vi "BackupPeriodicTasks.vi"() -> ()   [LabVIEW 2014]
uses:
  <vilib>/Rock Robotics/WPI/Joystick/WPI_JoystickGetSetRefNum.vi
  SwerveCode/SteerGlobals.vi
  <vilib>/addons/control/pid/pid.llb/PID (DBL).vi
  <vilib>/addons/control/pid/NI_PID_pid.lvlib
panel:
  in  "PID gains":T1={"proportional gain (Kc)"=0.0017, "integral time (Ti, min)"=0.01, "derivative time (Td, min)"=0.00173} {"derivative time (Td, min)" format="%.5f"; "integral time (Ti, min)" format="%.3f"; "proportional gain (Kc)" format="%.5f"}
  in  "error in":errorcluster
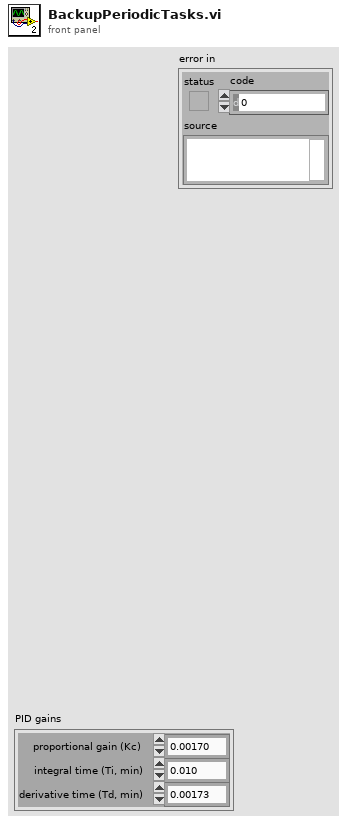
[diagram p1: front panel]
types:
  T1 = cluster{"proportional gain (Kc)":dbl, "integral time (Ti, min)":dbl, "derivative time (Td, min)":dbl}
  T2 = typedef "WPI_MotorControlDeviceRef.ctl" = cluster{"DeviceStatus":errorcluster, "Type":T3, "PWM":cluster{"Controller":T4, "PWM Channel":T5, "DeadBand":T6}, "CAN":cluster{"Device Number":u8, "Control Mode":T7, "Semaphore":T8, "Max Vout":dbl, "TalonSRX Control Mode":T9}, "Invert":bool, "TransformRef":T10, "InvTransformRef":T10}
  T3 = typedef "WPI_MotorControlType.ctl" = enum16{"PWM", "CAN", "CANTalonSRX"}
  T4 = typedef "FPGA_TypedefDigitalModule.ctl" = enum16{"Controller 1"}
  T5 = typedef "FPGA_DIOPWMChannel.ctl" = enum8{"PWM 0", "PWM 1", "PWM 2", "PWM 3", "PWM 4", "PWM 5", "PWM 6", "PWM 7", "PWM 8", "PWM 9", "PWM MXP 0", "PWM MXP 1", "PWM MXP 2", "PWM MXP 3", "PWM MXP 4", "PWM MXP 5", "PWM MXP 6", "PWM MXP 7", "PWM MXP 8", "PWM MXP 9", "Invalid"}
  T6 = typedef "WPI_PWMDeadband.ctl" = cluster{"Name":string, "maxPositivePwm":i32, "minPositivePwm":i32, "centerPwm":i32, "maxNegativePwm":i32, "minNegativePwm":i32, "angularRange":u16}
  T7 = typedef "WPI_CANJaguar_ControlMode.ctl" = enum8{"Percent VBus", "Current", "Speed", "Position", "Voltage"}
  T8 = typedef "Semaphore RefNum" = refnum<k1>
  T9 = typedef "WPI_CANTalonSRX_APIControlMode.ctl" = enum8{"Percent VBus", "Speed", "Position", "Slave", "Unchanged / Invalid"}
  T10 = typedef "WPI_PWMTransform_ConPane.ctl" = refnum<vi>
  T11 = typedef "WPI_JoystickDevRef.ctl" = cluster{"Device":T12}
  T12 = typedef "WPI_JoystickDeviceEnum.ctl" = enum16{"USB 0", "USB 1", "USB 2", "USB 3", "USB 4", "USB 5"}
  T13 = typedef "WPI_CANTalonSRX_GlobalStatus.ctl" = cluster{"Applied Throttle":dbl, "Module Enabled":bool, "CAN Error":errorcluster, "Closed Loop Error":dbl, "Forward Limit Switch Closed":bool, "Reverse Limit Switch Closed":bool, "Sensor Position":dbl, "Sensor Velocity":dbl, "Current":dbl, "Sticky Fault - Over Temp":bool, "Sticky Fault - Under Voltage":bool, "Sticky Fault - Forward Limit":bool, "Sticky Fault - Reverse Limit":bool, "Sticky Fault - Forward Soft Limit":bool, "Sticky Fault - Reverse Soft Limit":bool, "Brake is Enabled":bool, "Encoder Position":dbl, "Encoder Velocity":dbl, "Encoder Index Count":dbl, "Encoder A Pin State":bool, "Encoder B Pin State":bool, "Encoder Index Pin State":bool, "Analog In":dbl, "Analog In Velocity":dbl, "Temperature (C)":dbl, "Battery Voltage":dbl}
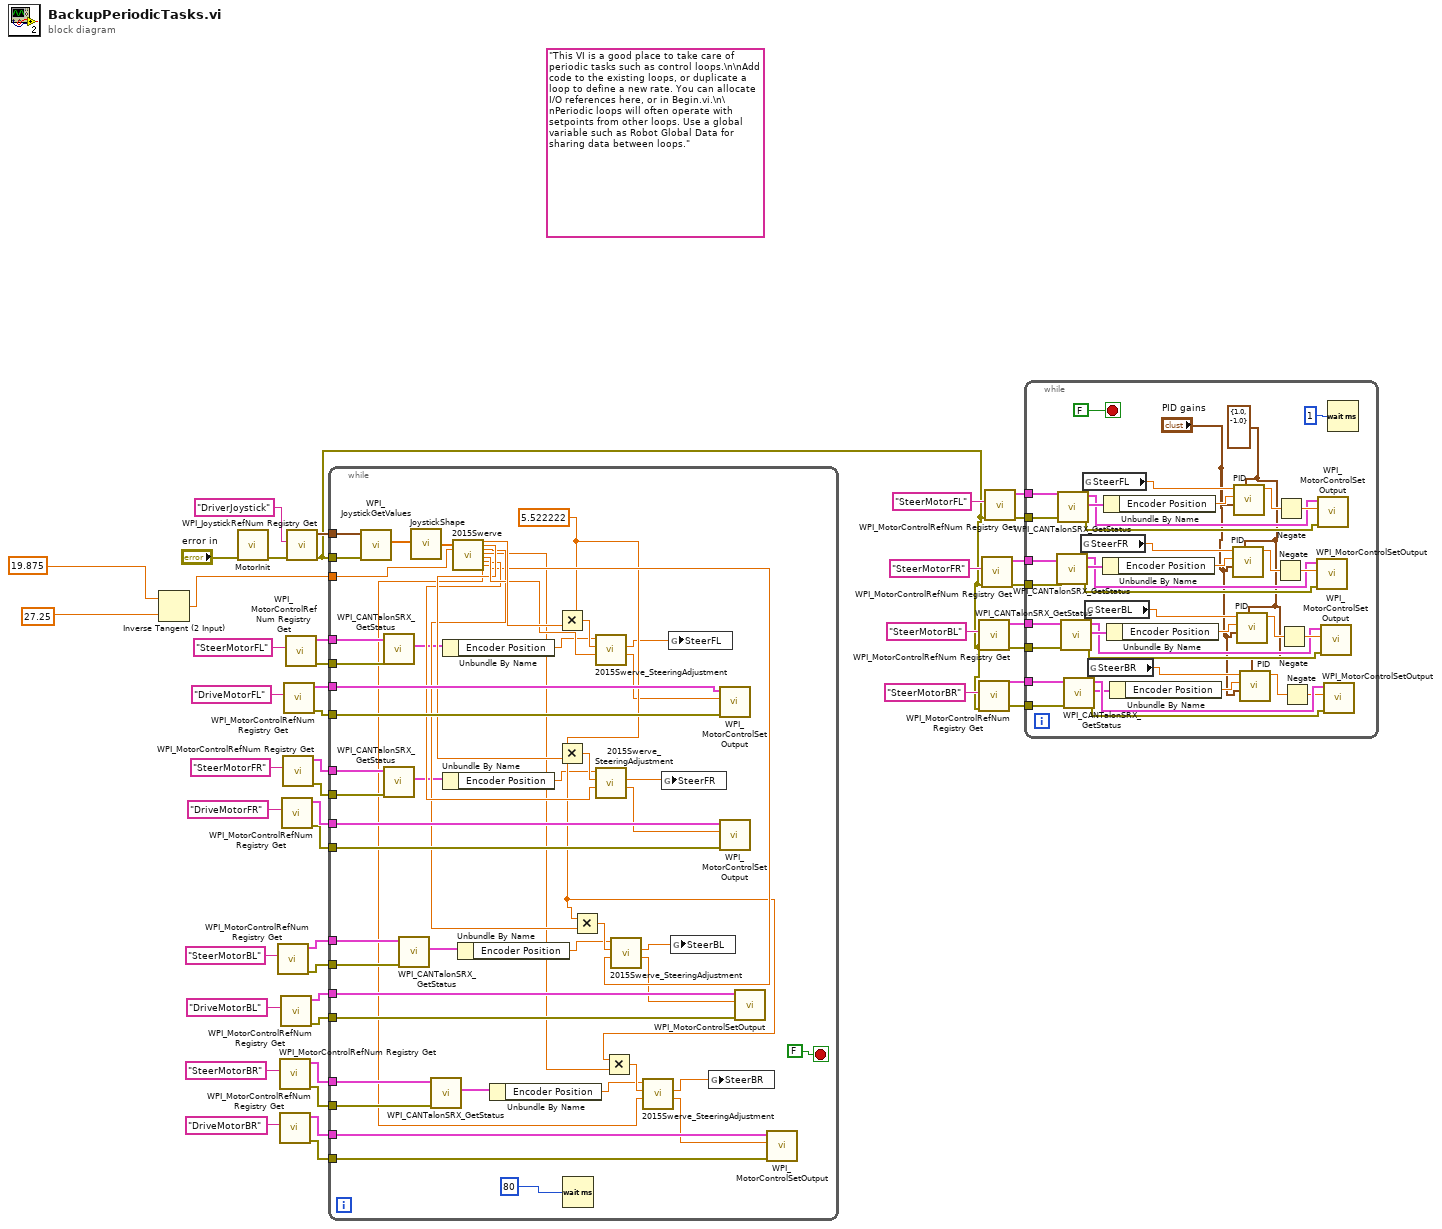
[diagram p0: block diagram]
diagram:
  (unwired) "This VI is a good place to take care of periodic tasks such as control loops.\n\nAdd code to the existing loops, or duplicate a loop to define a new rate. You can allocate I/O references here, or in Begin.vi.\n\nPeriodic loops will often operate with setpoints from other loops. Use a global variable such as Robot Global Data for sharing data between loops."
  n1 = Inverse Tangent (2 Input)(1:27.25 ("Robot Width"), 2:19.875 ("Robot Length")) -> (0:w2:dbl)
  n2 = call "MotorInit.vi"("error in"="error in") -> ("error out"=w41:errorcluster)  [unwired: 10 in]
  n3 = call <vilib>:"WPI_MotorControlRefNum Registry Get.vi"("refnum name"="SteerMotorBL") -> ("error out"=w24:errorcluster, "MotorControlDevRef"=w25:T2)  [unwired: 9 in]
  n4 = call <vilib>:"WPI_MotorControlRefNum Registry Get.vi"("refnum name"="SteerMotorBR") -> ("error out"=w19:errorcluster, "MotorControlDevRef"=w20:T2)  [unwired: 9 in]
  n5 = call <vilib>:"WPI_MotorControlRefNum Registry Get.vi"("refnum name"="DriveMotorBR") -> ("error out"=w17:errorcluster, "MotorControlDevRef"=w18:T2)  [unwired: 9 in]
  n6 = call <vilib>:"WPI_MotorControlRefNum Registry Get.vi"("refnum name"="DriveMotorBL") -> ("error out"=w21:errorcluster, "MotorControlDevRef"=w22:T2)  [unwired: 9 in]
  n7 = call <vilib>:"WPI_MotorControlRefNum Registry Get.vi"("refnum name"="DriveMotorFR") -> ("error out"=w26:errorcluster, "MotorControlDevRef"=w27:T2)  [unwired: 9 in]
  n8 = call <vilib>:"WPI_MotorControlRefNum Registry Get.vi"("refnum name"="SteerMotorFR") -> ("error out"=w28:errorcluster, "MotorControlDevRef"=w29:T2)  [unwired: 9 in]
  n9 = call <vilib>:"WPI_MotorControlRefNum Registry Get.vi"("refnum name"="DriveMotorFL") -> ("error out"=w30:errorcluster, "MotorControlDevRef"=w31:T2)  [unwired: 9 in]
  n10 = call <vilib>:"WPI_MotorControlRefNum Registry Get.vi"("refnum name"="SteerMotorFL") -> ("error out"=w32:errorcluster, "MotorControlDevRef"=w33:T2)  [unwired: 9 in]
  n11 = call <vilib>:"WPI_JoystickRefNum Registry Get.vi"("error in (no error)"=w41, "refnum name"="DriverJoystick") -> ("error out"=w1:errorcluster, "JoystickDevRef"=w42:T11)  [unwired: 8 in]
  n12 = while {
    tunnel: w42 -> [w94]
    tunnel: w1 -> [w93]
    tunnel: w33 -> [w92]
    tunnel: w32 -> [w91]
    tunnel: w31 -> [w88]
    tunnel: w30 -> [w87]
    tunnel: w29 -> [w84]
    tunnel: w28 -> [w83]
    tunnel: w27 -> [w82]
    tunnel: w26 -> [w81]
    tunnel: w25 -> [w78]
    tunnel: w24 -> [w77]
    tunnel: w22 -> [w76]
    tunnel: w21 -> [w75]
    tunnel: w20 -> [w74]
    tunnel: w19 -> [w73]
    tunnel: w18 -> [w72]
    tunnel: w17 -> [w71]
    tunnel: w2 -> [w45]
    stop <- FALSE stop-if-true
    w69 = 5.522222 ("y")
    n13 = call <vilib>:"WPI_JoystickGetValues.vi"("error in (no error)"=w93, "JoystickDevRef"=w94) -> ("Axes"=w47:dbl[])  [unwired: 5 in, 4 out]
    n14 = call <vilib>:"WPI_CANTalonSRX_GetStatus.vi"("error in (no error)"=w91, "CAN Talon SRX Ref"=w92) -> ("Talon SRX Status"=w67:T13)  [unwired: 7 in, 2 out]
    n15 = call <vilib>:"WPI_CANTalonSRX_GetStatus.vi"("error in (no error)"=w83, "CAN Talon SRX Ref"=w84) -> ("Talon SRX Status"=w63:T13)  [unwired: 7 in, 2 out]
    n16 = call <vilib>:"WPI_CANTalonSRX_GetStatus.vi"("error in (no error)"=w77, "CAN Talon SRX Ref"=w78) -> ("Talon SRX Status"=w59:T13)  [unwired: 7 in, 2 out]
    n17 = call "JoystickShape.vi"("JoystickValues"=w47) -> ("appended array"=w46:dbl[])
    n18 = call <vilib>:"WPI_CANTalonSRX_GetStatus.vi"("error in (no error)"=w73, "CAN Talon SRX Ref"=w74) -> ("Talon SRX Status"=w55:T13)  [unwired: 7 in, 2 out]
    n19 = Unbundle By Name(w67) -> ("Encoder Position"=w65:dbl)
    n20 = Unbundle By Name(w63) -> ("Encoder Position"=w61:dbl)
    n21 = call "2015Swerve.vi"("Axes"=w46, "Robot Dimension Calc"=w45) -> ("FL Angle"=w90:dbl, "FR Angle"=w86:dbl, "BL Angle"=w80:dbl, "BR Angle"=w70:dbl, "FL Power"=w89:dbl, "FR Power"=w85:dbl, "BL Power"=w79:dbl, "BR Power"=w68:dbl)  [unwired: 18 in]
    n22 = Unbundle By Name(w59) -> ("Encoder Position"=w57:dbl)
    n23 = Unbundle By Name(w55) -> ("Encoder Position"=w53:dbl)
    n24 = Multiply(x=w69, y=w90) -> (x*y=w66:dbl)
    n25 = Multiply(x=w69, y=w86) -> (x*y=w62:dbl)
    n26 = Wait (ms)(milliseconds to wait=u32 80) -> ()  [unwired: 1 out]
    n27 = Multiply(x=w69, y=w80) -> (x*y=w58:dbl)
    n28 = call "2015Swerve_SteeringAdjustment.vi"("Wheel Power"=w89, "Encoder Setpoint"=w66, "Encoder Position"=w65) -> ("Wheel Power Out"=w64:dbl, "Encoder Setpoint Out"=w51:dbl)  [unwired: 7 in]
    n29 = call "2015Swerve_SteeringAdjustment.vi"("Wheel Power"=w85, "Encoder Setpoint"=w62, "Encoder Position"=w61) -> ("Wheel Power Out"=w60:dbl, "Encoder Setpoint Out"=w50:dbl)  [unwired: 7 in]
    n30 = Multiply(x=w69, y=w70) -> (x*y=w54:dbl)
    n31 = call "2015Swerve_SteeringAdjustment.vi"("Wheel Power"=w79, "Encoder Setpoint"=w58, "Encoder Position"=w57) -> ("Wheel Power Out"=w56:dbl, "Encoder Setpoint Out"=w49:dbl)  [unwired: 7 in]
    n32 = call "2015Swerve_SteeringAdjustment.vi"("Wheel Power"=w68, "Encoder Setpoint"=w54, "Encoder Position"=w53) -> ("Wheel Power Out"=w52:dbl, "Encoder Setpoint Out"=w48:dbl)  [unwired: 7 in]
    n33 = global write "SteerGlobals.vi" "SteerFR"(w50) -> ()
    n34 = global write "SteerGlobals.vi" "SteerFL"(w51) -> ()
    n35 = global write "SteerGlobals.vi" "SteerBL"(w49) -> ()
    n36 = global write "SteerGlobals.vi" "SteerBR"(w48) -> ()
    n37 = call <vilib>:"WPI_MotorControlSetOutput.vi"("error in (no error)"=w87, "Output"=w64, "MotorControlDevRef"=w88) -> ()  [unwired: 6 in, 3 out]
    n38 = call <vilib>:"WPI_MotorControlSetOutput.vi"("error in (no error)"=w81, "Output"=w60, "MotorControlDevRef"=w82) -> ()  [unwired: 6 in, 3 out]
    n39 = call <vilib>:"WPI_MotorControlSetOutput.vi"("error in (no error)"=w75, "Output"=w56, "MotorControlDevRef"=w76) -> ()  [unwired: 6 in, 3 out]
    n40 = call <vilib>:"WPI_MotorControlSetOutput.vi"("error in (no error)"=w71, "Output"=w52, "MotorControlDevRef"=w72) -> ()  [unwired: 6 in, 3 out]
  }
  n41 = call <vilib>:"WPI_MotorControlRefNum Registry Get.vi"("error in (no error)"=w1, "refnum name"="SteerMotorBL") -> ("error out"=w7:errorcluster, "MotorControlDevRef"=w8:T2)  [unwired: 8 in]
  n42 = call <vilib>:"WPI_MotorControlRefNum Registry Get.vi"("error in (no error)"=w1, "refnum name"="SteerMotorBR") -> ("error out"=w5:errorcluster, "MotorControlDevRef"=w6:T2)  [unwired: 8 in]
  n43 = call <vilib>:"WPI_MotorControlRefNum Registry Get.vi"("error in (no error)"=w1, "refnum name"="SteerMotorFR") -> ("error out"=w9:errorcluster, "MotorControlDevRef"=w10:T2)  [unwired: 8 in]
  n44 = call <vilib>:"WPI_MotorControlRefNum Registry Get.vi"("error in (no error)"=w1, "refnum name"="SteerMotorFL") -> ("error out"=w11:errorcluster, "MotorControlDevRef"=w12:T2)  [unwired: 8 in]
  n45 = while {
    tunnel: w12 -> [w133]
    tunnel: w11 -> [w132]
    tunnel: w10 -> [w118]
    tunnel: w9 -> [w117]
    tunnel: w8 -> [w109]
    tunnel: w7 -> [w108]
    tunnel: w6 -> [w98]
    tunnel: w5 -> [w97]
    stop <- FALSE stop-if-true
    w99 = cluster{"output high":dbl, "output low":dbl} {"output high"=1.0, "output low"=-1.0} ("output range")
    n46 = call <vilib>:"WPI_CANTalonSRX_GetStatus.vi"("error in (no error)"=w117, "CAN Talon SRX Ref"=w118) -> ("error out"=w119:errorcluster, "Talon SRX Status"=w124:T13, "CAN Talon SRX Ref Out"=w120:T2)  [unwired: 7 in]
    n47 = call <vilib>:"WPI_CANTalonSRX_GetStatus.vi"("error in (no error)"=w132, "CAN Talon SRX Ref"=w133) -> ("error out"=w126:errorcluster, "Talon SRX Status"=w131:T13, "CAN Talon SRX Ref Out"=w127:T2)  [unwired: 7 in]
    n48 = call <vilib>:"WPI_CANTalonSRX_GetStatus.vi"("error in (no error)"=w108, "CAN Talon SRX Ref"=w109) -> ("error out"=w110:errorcluster, "Talon SRX Status"=w115:T13, "CAN Talon SRX Ref Out"=w111:T2)  [unwired: 7 in]
    n49 = call <vilib>:"WPI_CANTalonSRX_GetStatus.vi"("error in (no error)"=w97, "CAN Talon SRX Ref"=w98) -> ("error out"=w107:errorcluster, "Talon SRX Status"=w102:T13, "CAN Talon SRX Ref Out"=w106:T2)  [unwired: 7 in]
    n50 = global read "SteerGlobals.vi" "SteerFR"() -> (w125:dbl)
    n51 = global read "SteerGlobals.vi" "SteerFL"() -> (w134:dbl)
    n52 = global read "SteerGlobals.vi" "SteerBL"() -> (w116:dbl)
    n53 = global read "SteerGlobals.vi" "SteerBR"() -> (w101:dbl)
    n54 = Unbundle By Name(w124) -> ("Encoder Position"=w123:dbl)
    n55 = Unbundle By Name(w131) -> ("Encoder Position"=w130:dbl)
    n56 = Unbundle By Name(w115) -> ("Encoder Position"=w114:dbl)
    n57 = Unbundle By Name(w102) -> ("Encoder Position"=w103:dbl)
    n58 = call-poly <vilib>:"PID.vi"("output range"=w99, "PID gains"="PID gains", "process variable"=w123, "setpoint"=w125) -> ("output"=w122:dbl)  [unwired: 6 in, 1 out]
    n59 = call-poly <vilib>:"PID.vi"("output range"=w99, "PID gains"="PID gains", "process variable"=w130, "setpoint"=w134) -> ("output"=w129:dbl)  [unwired: 6 in, 1 out]
    n60 = call-poly <vilib>:"PID.vi"("output range"=w99, "PID gains"="PID gains", "process variable"=w114, "setpoint"=w116) -> ("output"=w113:dbl)  [unwired: 6 in, 1 out]
    n61 = call-poly <vilib>:"PID.vi"("output range"=w99, "PID gains"="PID gains", "process variable"=w103, "setpoint"=w101) -> ("output"=w104:dbl)  [unwired: 6 in, 1 out]
    n62 = Negate(x=w122) -> (-x=w121:dbl)
    n63 = Negate(x=w129) -> (-x=w128:dbl)
    n64 = Negate(x=w113) -> (-x=w112:dbl)
    n65 = Negate(x=w104) -> (-x=w105:dbl)
    n66 = call <vilib>:"WPI_MotorControlSetOutput.vi"("error in (no error)"=w119, "Output"=w121, "MotorControlDevRef"=w120) -> ()  [unwired: 6 in, 3 out]
    n67 = call <vilib>:"WPI_MotorControlSetOutput.vi"("error in (no error)"=w126, "Output"=w128, "MotorControlDevRef"=w127) -> ()  [unwired: 6 in, 3 out]
    n68 = call <vilib>:"WPI_MotorControlSetOutput.vi"("error in (no error)"=w110, "Output"=w112, "MotorControlDevRef"=w111) -> ()  [unwired: 6 in, 3 out]
    n69 = call <vilib>:"WPI_MotorControlSetOutput.vi"("error in (no error)"=w107, "Output"=w105, "MotorControlDevRef"=w106) -> ()  [unwired: 6 in, 3 out]
    n70 = Wait (ms)(milliseconds to wait=u32 1) -> ()  [unwired: 1 out]
  }
